vi "Joint Reference Follower (beta).vi"(6 "Accurus Ctrl Cluster":T2={"Stop Vacuum"=TRUE, "Vacuum Force"=0, "Max Limit [mmHg]"=600.0, "Slide in"=0, "Irrigation?"=TRUE} {"Slide in" scale=0.0..78.0; "Vacuum Force" min=0 max=78}, 7 "Offset Home2RCM [deg/mm]":dbl[](array[numeric])=[0.0, 0.0, 0.0, 0.0], 8 "PID Ctrl Cluster":T3={"L1 PID Gains"={"Kp"=0.005, "Kd"=0.5, "Ki"=0.0005}, "L2 PID Gains"={"Kp"=0.01, "Kd"=1.0, "Ki"=0.005}, "L3 PID Gains"={"Kp"=0.05, "Kd"=1.0, "Ki"=0.0005}, "L4 PID Gains"={"Kp"=0.1, "Kd"=0.1, "Ki"=0.0005}}, 9 "Ref Array [deg/mm]":dbl[](array[numeric])=[0.0, 0.0, 0.0, 0.0], 10 "error in":errorcluster, 11 "FPGA VI Reference In":refnum<k20>) -> (0 "Accurus Output Cluster":T1, 1 "Output Posit Array [deg/mm]":dbl[](array[numeric]), 2 "error out":errorcluster, 3 "FPGA VI Reference Out":refnum<k20>)   [LabVIEW 2016]
uses:
  <vilib>/rvi/errors/niLvFpgaAdjustHostInterfaceError.vi
  <vilib>/Utility/error.llb/Error Cluster From Error Code.vi
  Subsystems/Global Variables.vi
  <vilib>/rvi/interface/nirviReadWriteControl/nirviReadWriteControl.xnode
  FPGA Bitfiles/PhantomControlPI_FPGATarget_QuadCtr2_E2412E44.lvbitx
  IRISS_FPGA_IO.vi
  Library/KevinLibraryAll/labview/KevLib01.lvlib
  NiFpgaLv.dll
panel:
  # "button 1"
  # "button 2"
  # "button 3"
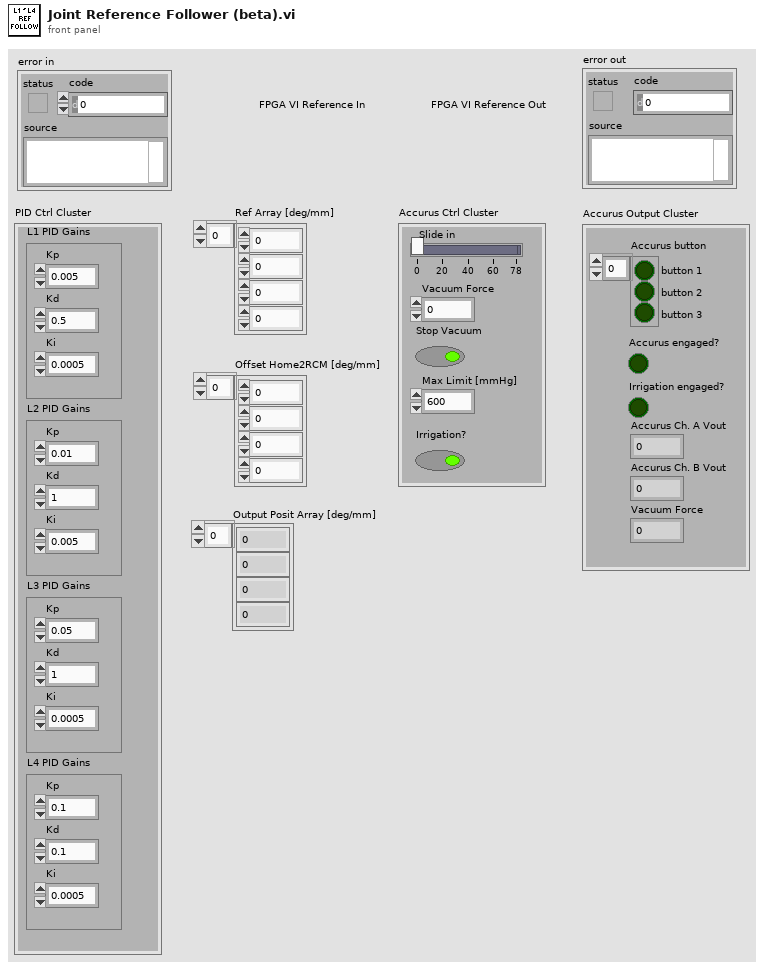
[diagram p1: front panel]
types:
  T1 = cluster{"Accurus button":bool[], "Accurus engaged?":bool, "Vacuum Force":i32, "Accurus Ch. A Vout":dbl, "Accurus Ch. B Vout":dbl, "Irrigation engaged?":bool}
  T2 = cluster{"Stop Vacuum":bool, "Vacuum Force":i8, "Max Limit [mmHg]":dbl, "Slide in":i8, "Irrigation?":bool}
  T3 = cluster{"L1 PID Gains":cluster{"Kp":dbl, "Kd":dbl, "Ki":dbl}, "L2 PID Gains":cluster{"Kp":dbl, "Kd":dbl, "Ki":dbl}, "L3 PID Gains":cluster{"Kp":dbl, "Kd":dbl, "Ki":dbl}, "L4 PID Gains":cluster{"Kp":dbl, "Kd":dbl, "Ki":dbl}}
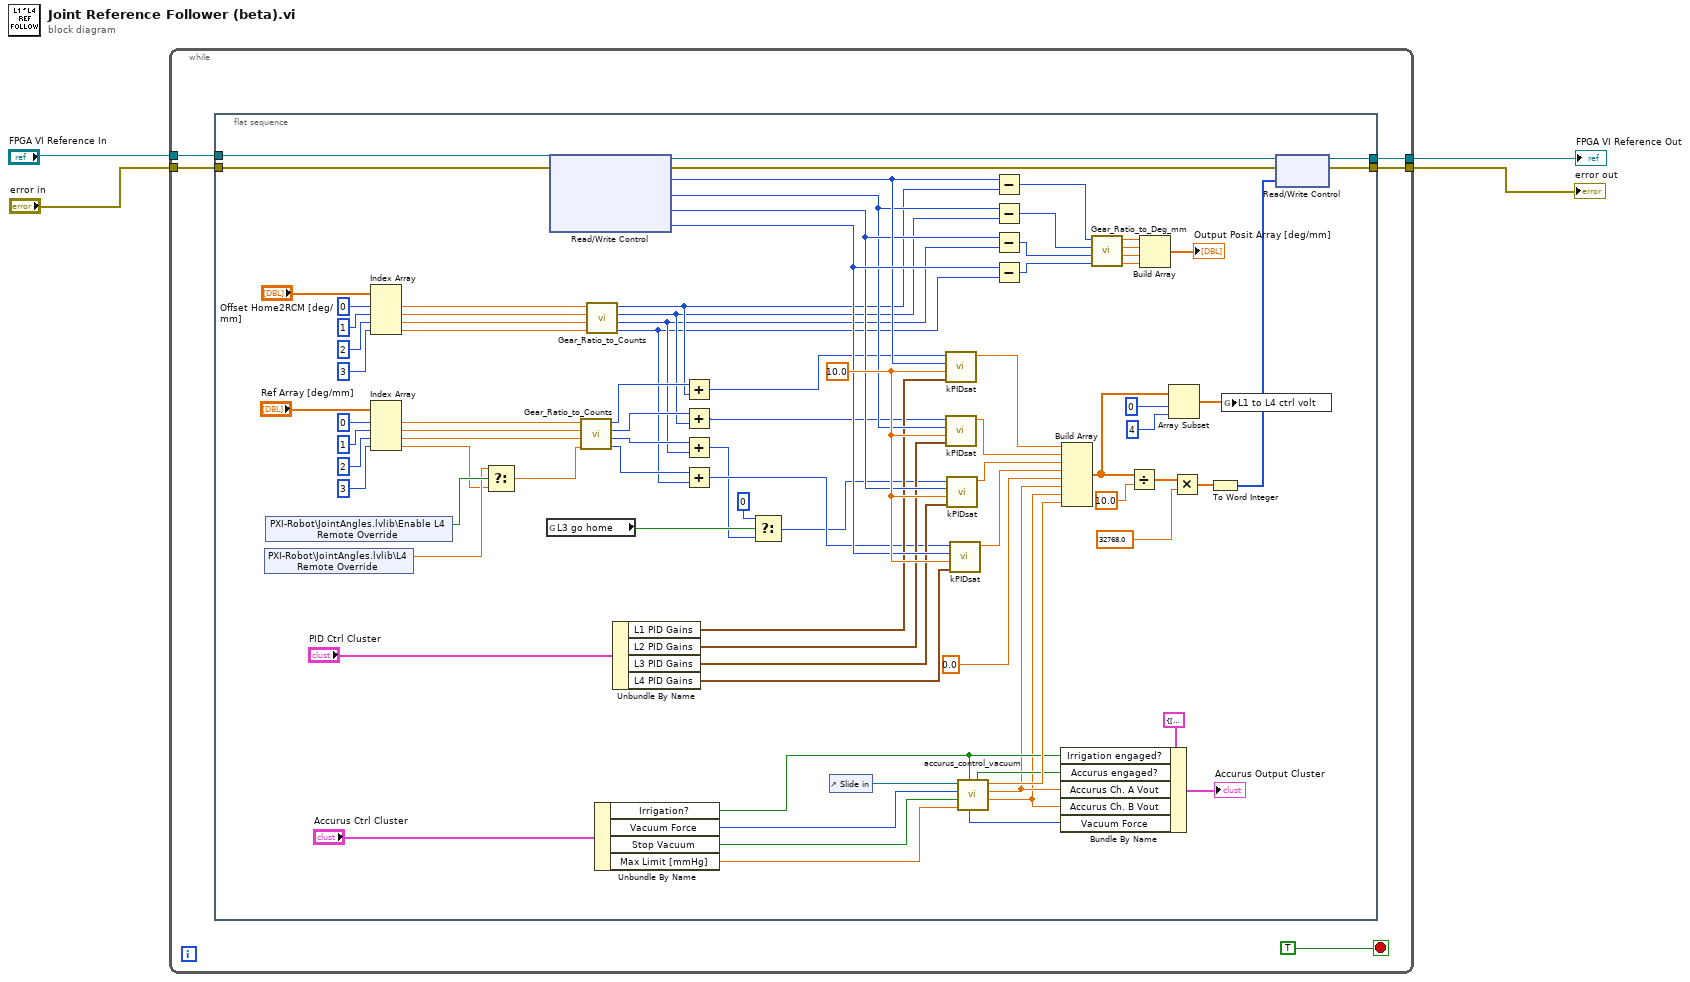
[diagram p0: block diagram]
diagram:
  n1 = while {
    tunnel: [w9] -> w1
    tunnel: [w8] -> w4
    tunnel: "FPGA VI Reference In" -> [w7]
    tunnel: "error in" -> [w6]
    stop <- TRUE ("Boolean") stop-if-true
    n2 = flat-sequence {
      tunnel: [w74] -> w9
      tunnel: [w73] -> w8
      tunnel: w7 -> [w50]
      tunnel: w6 -> [w49]
      frame #0 {
        w83 = 10.0 ("Sat Limit")
        n3 = shared-variable "PXI-Robot\\JointAngles.lvlib\\L4 Remote Override"() -> (w23:dbl)  [unwired: 1 in, 1 out]
        n4 = shared-variable "PXI-Robot\\JointAngles.lvlib\\Enable L4 Remote Override"() -> (w24:bool)  [unwired: 1 in, 1 out]
        n5 = Index Array(array="Offset Home2RCM [deg/mm]", index #1=0 ("index"), index #2=1 ("index"), index #3=2 ("index"), index #4=3 ("index")) -> (element #1=w48:dbl, element #2=w47:dbl, element #3=w46:dbl, element #4=w45:dbl)
        n6 = Index Array(array="Ref Array [deg/mm]", index #1=0 ("index"), index #2=1 ("index"), index #3=2 ("index"), index #4=3 ("index")) -> (element #1=w91:dbl, element #2=w90:dbl, element #3=w89:dbl, element #4=w22:dbl)
        n7 = Select(t=w23, s=w24, f=w22) -> (s? t:f=w21:dbl)
        n8 = global read "Global Variables.vi" "L3 go home"() -> (w28:bool)
        n9 = xnode "Read/Write Control"("FPGA VI Reference In"=w50, "error in"=w49) -> ("FPGA VI Reference Out"=w76:refnum<k20>, "error out"=w75:errorcluster, "32 bit Position 1"=w57:i32, "32 bit Position 3"=w55:i32, "32 bit Position C1-1"=w56:i32, "32 bit Position C1-4"=w67:i32)
        n10 = call "Gear_Ratio_to_Counts.vi"("theta 4"=w21, "theta 3"=w89, "theta 2"=w90, "theta 1"=w91) -> ("j4"=w38:i32, "j3"=w39:i32, "j2"=w40:i32, "j1"=w41:i32)
        n11 = call "Gear_Ratio_to_Counts.vi"("theta 4"=w45, "theta 3"=w46, "theta 2"=w47, "theta 1"=w48) -> ("j4"=w34:i32, "j3"=w35:i32, "j2"=w36:i32, "j1"=w37:i32)
        n12 = Unbundle By Name("Accurus Ctrl Cluster") -> ("Irrigation?"=w19:bool, "Vacuum Force"=w32:i8, "Stop Vacuum"=w31:bool, "Max Limit [mmHg]"=w30:dbl)
        n13 = Unbundle By Name("PID Ctrl Cluster") -> ("L1 PID Gains"=w54:cluster{"Kp":dbl, "Kd":dbl, "Ki":dbl}, "L2 PID Gains"=w53:cluster{"Kp":dbl, "Kd":dbl, "Ki":dbl}, "L3 PID Gains"=w52:cluster{"Kp":dbl, "Kd":dbl, "Ki":dbl}, "L4 PID Gains"=w51:cluster{"Kp":dbl, "Kd":dbl, "Ki":dbl})
        n14 = Add(x=w41, y=w37) -> (x+y=w44:i32)
        n15 = Add(x=w40, y=w36) -> (x+y=w43:i32)
        n16 = Add(x=w39, y=w35) -> (x+y=w27:i32)
        n17 = Add(x=w38, y=w34) -> (x+y=w42:i32)
        n18 = Select(t=0 ("index"), s=w28, f=w27) -> (s? t:f=w25:i32)
        n19 = control-ref of="Slide in"() -> (w29:refnum<vi>)
        n20 = call "kPIDsat.vi"("PID Gains"=w54, "Sat Limit"=w83, "Position"=w57, "Reference"=w44) -> ("Control"=w66:dbl)  [unwired: 7 in]
        n21 = call "kPIDsat.vi"("PID Gains"=w53, "Sat Limit"=w83, "Position"=w55, "Reference"=w43) -> ("Control"=w68:dbl)  [unwired: 7 in]
        n22 = call "kPIDsat.vi"("PID Gains"=w52, "Sat Limit"=w83, "Position"=w56, "Reference"=w25) -> ("Control"=w69:dbl)  [unwired: 7 in]
        n23 = call "kPIDsat.vi"("PID Gains"=w51, "Sat Limit"=w83, "Position"=w67, "Reference"=w42) -> ("Control"=w82:dbl)  [unwired: 7 in]
        n24 = call "accurus_control_vacuum.vi"("Irrigate?"=w19, "Max Limit [mmHg]"=w30, "stop"=w31, "vacuum force"=w32, "Slide in"=w29) -> ("f"=w16:dbl, "f 2"=w17:dbl, "f 3"=w71:dbl, "Boolean 2"=w18:bool, "Vacuum Force\n[mmHg]"=w15:i32)  [unwired: 1 in, 1 out]
        n25 = Subtract(x=w57, y=w37) -> (x-y=w61:i32)
        n26 = Subtract(x=w55, y=w36) -> (x-y=w60:i32)
        n27 = Subtract(x=w56, y=w35) -> (x-y=w59:i32)
        n28 = Subtract(x=w67, y=w34) -> (x-y=w58:i32)
        n29 = Bundle By Name(cluster=T1 {"Accurus button"=[FALSE, FALSE, FALSE], "Accurus engaged?"=FALSE, "Vacuum Force"=0, "Accurus Ch. A Vout"=0.0, "Accurus Ch. B Vout"=0.0, "Irrigation engaged?"=FALSE} ("Accurus Output Cluster"), "Irrigation engaged?"=w19, "Accurus engaged?"=w18, "Accurus Ch. A Vout"=w17, "Accurus Ch. B Vout"=w16, "Vacuum Force"=w15) -> (→"Accurus Output Cluster":T1)
        n30 = Build Array(w66, w68, w69, w82, 0.0 ("element"), w17, w16, w71) -> (w13:dbl[])
        n31 = call "Gear_Ratio_to_Deg_mm.vi"("j4"=w58, "j3"=w59, "j2"=w60, "j1"=w61) -> ("theta 4"=w62:dbl, "theta 3"=w63:dbl, "theta 2"=w64:dbl, "theta 1"=w65:dbl)
        n32 = Divide(x=w13, y=10.0) -> (x/y=w80:dbl[])
        n33 = Build Array(w65, w64, w63, w62) -> (→"Output Posit Array [deg/mm]":dbl[])
        n34 = Array Subset(array=w13, index=0, length=4) -> (w10:dbl[])
        n35 = Multiply(x=w80, y=32768.0) -> (x*y=w78:dbl[])
        n36 = To Word Integer(number=w78) -> (16bit integer=w77:i16[])
        n37 = global write "Global Variables.vi" "L1 to L4 ctrl volt"(w10) -> ()
        n38 = xnode "Read/Write Control"("FPGA VI Reference In"=w76, "error in"=w75, "AO"=w77) -> ("FPGA VI Reference Out"=w74:refnum<k20>, "error out"=w73:errorcluster)
      }
    }
  }
  "error out" <- w4
  "FPGA VI Reference Out" <- w1
